vi "Operator Loop OLD.vi"() -> ()   [LabVIEW 2011]
uses:
  <vilib>/Platform/TimedLoop/XDataNode/timing_clust.ctl
  <vilib>/Platform/TimedLoop/XDataNode/nitl_modes.ctl
  <vilib>/Platform/TimedLoop/XDataNode/wakeup.ctl
  <vilib>/Platform/TimedLoop/XDataNode/XDataNode.xnode
  <vilib>/Platform/TimedLoop/XDataNode/XDNodeRunTimeDep.lvlib
panel:
  out "Heading_Cmd":dbl
  out "VTan_Cmd":dbl
  out "VAng_Cmd":dbl
  in  "End Loop":bool
  out "Error Out":errorcluster
  in  "Error In":errorcluster
  in  "SubGoal Threshold":dbl=1.1
  in  "GPS Data":T1
  in  "IMU Data":T2
  in  "A star":bool=TRUE
  in  "outer threshold":dbl=1.1
  in  "inner threshold":dbl=0.6
  in  "max speed":dbl=0.4
  in  "stop?":bool
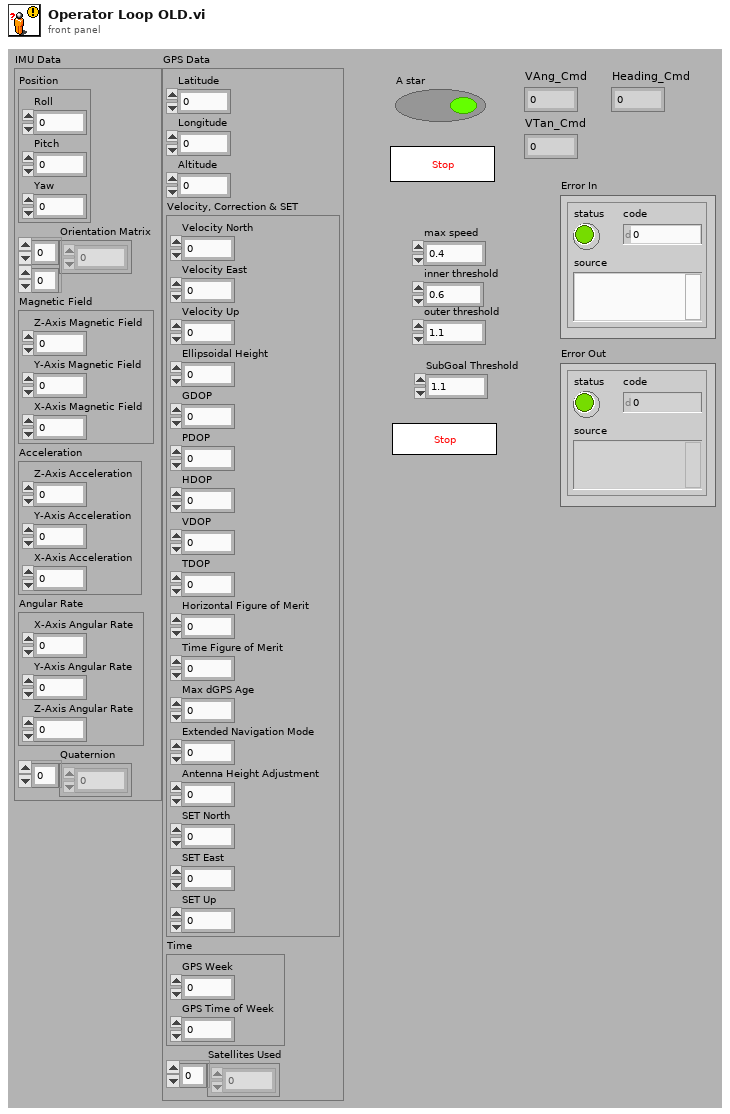
[diagram p1: front panel]
types:
  T1 = cluster{"Latitude":dbl, "Longitude":dbl, "Altitude":dbl, "Velocity, Correction & SET":cluster{"Velocity North":dbl, "Velocity East":dbl, "Velocity Up":dbl, "Ellipsoidal Height":dbl, "GDOP":sgl, "PDOP":sgl, "HDOP":sgl, "VDOP":sgl, "TDOP":sgl, "Horizontal Figure of Merit":u8, "Time Figure of Merit":u8, "Max dGPS Age":sgl, "Extended Navigation Mode":u8, "Antenna Height Adjustment ":dbl, "SET North":i32, "SET East":i32, "SET Up":i32}, "Time":cluster{"GPS Week":u16, "GPS Time of Week":sgl}, "Satellites Used":i32[]}
  T2 = cluster{"Position":cluster{"Roll":dbl, "Pitch":dbl, "Yaw":dbl}, "Orientation Matrix":dbl[][], "Magnetic Field":cluster{"Z-Axis Magnetic Field":dbl, "Y-Axis Magnetic Field":dbl, "X-Axis Magnetic Field":dbl}, "Acceleration":cluster{"Z-Axis Acceleration":dbl, "Y-Axis Acceleration":dbl, "X-Axis Acceleration":dbl}, "Angular Rate":cluster{"X-Axis Angular Rate":dbl, "Y-Axis Angular Rate":dbl, "Z-Axis Angular Rate":dbl}, "Quaternion":dbl[]}
  T3 = enum16{"Idle", "Wiimote", "Joypad", "IGVC", "Avoide Objects", "Avoide Lines", "Path Planning", "Heading", "Waypoint"}
  T4 = typedef "XDNodeRunTimeDep.lvlib/timing_clust.ctl" = cluster{"Expected End [f-1]":u64, "Actual End [f-1]":u64, "Finished Late? [f-1]":bool, "Expected End [i-1]":u64, "Actual End [i-1]":u64, "Finished Late? [i-1]":bool, "Expected Start [i]":u64, "Actual Start [i]":u64, "Expected Start [f]":u64, "Actual Start [f]":u64, "Source Name":string, "Structure Name":string, "Period":i64, "Deadline":i64, "Offset":i64, "Start":i64, "Priority":i32, "Timeout":i32, "Mode":T5, "Wakeup Reason":T6, "Error":errorcluster, "Source Type":string, "Secondary Source Type":string, "Global End Time":u64, "Global Start Time":u64, "Frame Duration":u64, "Iteration Duration":u64, "Assigned CPU":i32, "I/O Scan Engine Mode":u32}
  T5 = typedef "XDNodeRunTimeDep.lvlib/nitl_modes.ctl" = enum32{"No Change", "Process missed periods, maintain original phase", "Discard missed periods, maintain original phase", "Process missed periods, ignore original phase", "Discard missed periods, ignore original phase"}
  T6 = typedef "XDNodeRunTimeDep.lvlib/wakeup.ctl" = enum32{"Normal", "Aborted", "Asynchronous wakeup", "Timing source error", "Timed loop error", "Timeout"}
  T7 = cluster{"SubGoal":cluster{"Latitude":dbl, "Longitude":dbl, "Altitude":dbl, "Velocity, Correction & SET":cluster{"Velocity North":dbl, "Velocity East":dbl, "Velocity Up":dbl, "Ellipsoidal Height":dbl, "GDOP":sgl, "PDOP":sgl, "HDOP":sgl, "VDOP":sgl, "TDOP":sgl, "Horizontal Figure of Merit":u8, "Time Figure of Merit":u8, "Max dGPS Age":sgl, "Extended Navigation Mode":u8, "Antenna Height Adjustment ":dbl, "SET North":i32, "SET East":i32, "SET Up":i32}, "Time":cluster{"GPS Week":u16, "GPS Time of Week":sgl}, "Satellites Used":i32[]}, "Sub Goal Name":string}[]
  T8 = cluster{"SubGoal":cluster{"Latitude":dbl, "Longitude":dbl, "Altitude":dbl, "Velocity, Correction & SET":cluster{"Velocity North":dbl, "Velocity East":dbl, "Velocity Up":dbl, "Ellipsoidal Height":dbl, "GDOP":sgl, "PDOP":sgl, "HDOP":sgl, "VDOP":sgl, "TDOP":sgl, "Horizontal Figure of Merit":u8, "Time Figure of Merit":u8, "Max dGPS Age":sgl, "Extended Navigation Mode":u8, "Antenna Height Adjustment ":dbl, "SET North":i32, "SET East":i32, "SET Up":i32}, "Time":cluster{"GPS Week":u16, "GPS Time of Week":sgl}, "Satellites Used":i32[]}, "Sub Goal Name":string}
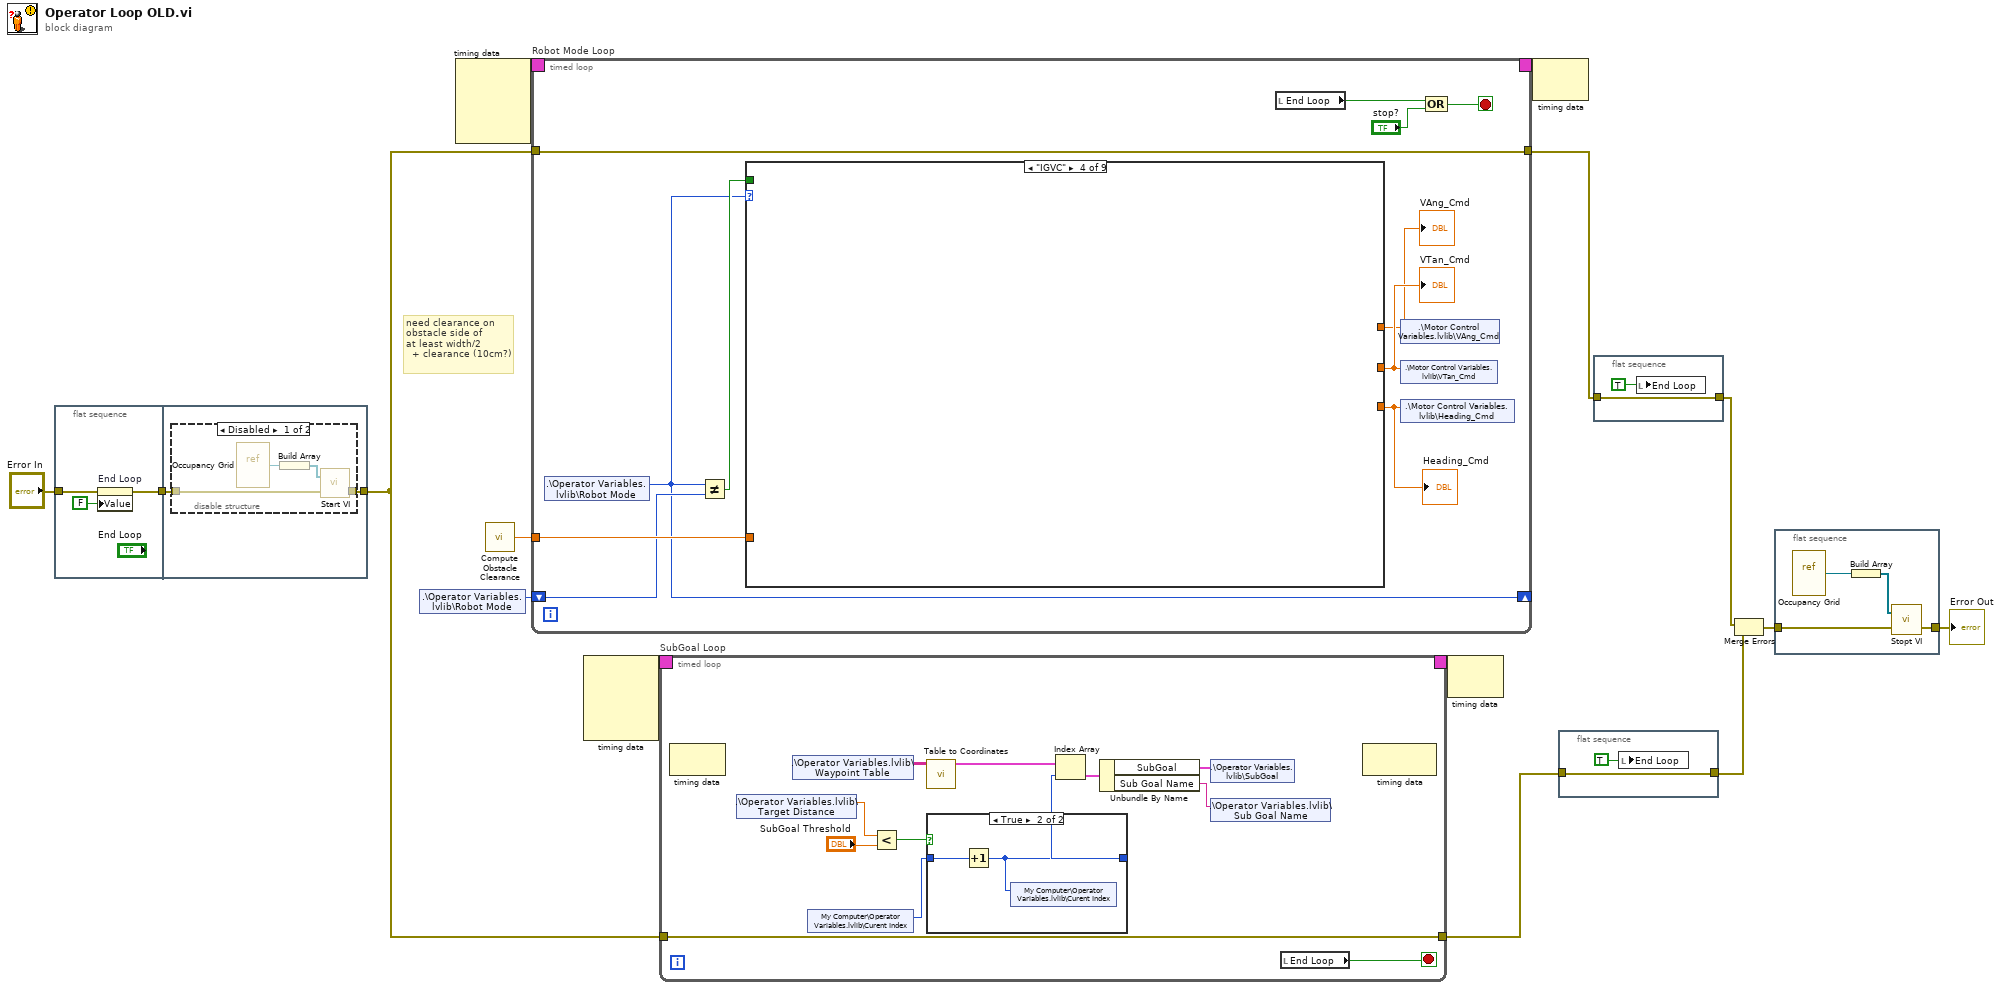
[diagram p0: block diagram]
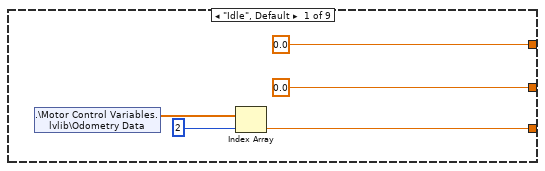
[diagram p4: hidden frame]
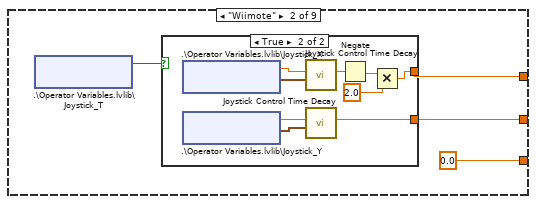
[diagram p5: hidden frame]
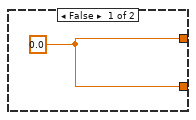
[diagram p6: hidden frame]
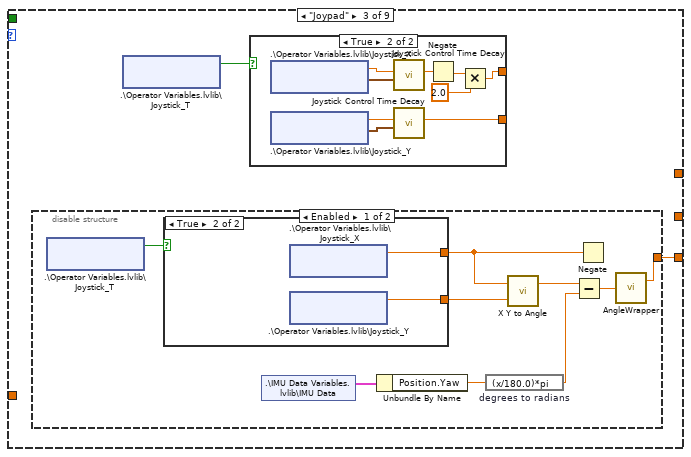
[diagram p7: hidden frame]
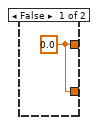
[diagram p8: hidden frame]
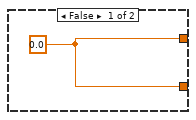
[diagram p10: hidden frame]
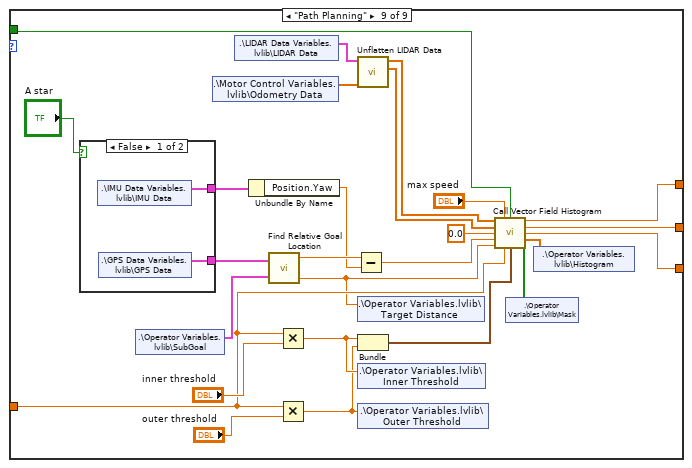
[diagram p15: hidden frame]
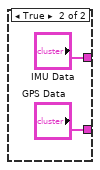
[diagram p16: hidden frame]
diagram:
  # "need clearance on \nobstacle side of \nat least width/2 \n  + clearance (10cm?)"
  n1 = flat-sequence {
    tunnel: "Error In" -> [w16]
    tunnel: [w17] -> w4
    tunnel: [w19] -> w5
    tunnel: w4 -> [w20]
    frame #0 {
      n2 = property on="End Loop" class="Bool (strict)"(error in=w16, "Value"=FALSE ("End Loop")) -> (error out=w17:errorcluster)  [unwired: 1 in, 1 out]
    }
    frame #1 {
      n3 = disable-structure shown="Disabled" {
        disable-tunnel: w20 -> [w22 w25]
        disable-tunnel: [w21 w25] -> w19
        frame Disabled {
          n4 = vi-ref "Occupancy Grid.vi"() -> (w24:refnum<vi>)
          n5 = Build Array(w24) -> (w23:refnum<vi>[])
          n6 = call "Start VI.vi"("error in"=w22, "VI refnum"=w23) -> ("error out"=w21:errorcluster)  [unwired: 1 in]
        }
        frame Enabled {
        }
      }
    }
  }
  n7 = shared-variable ".\\Operator Variables.lvlib\\Robot Mode"() -> (w12:T3)  [unwired: 1 in, 1 out]
  n8 = node-c288() -> (w15:T4)  [unwired: 4 in]
  n9 = call "Compute Obstacle Clearance.vi"() -> ("obstacle clearance (m)"=w13:dbl)  [unwired: 1 in]
  n10 = timed-loop "Robot Mode Loop" {
    timing: w15 -> [_]
    timing-out: [_] -> w14
    tunnel: w13 -> [w36]
    shift-right: [w33] -> _
    shift-left: w12 -> [w34]
    tunnel: w5 -> [w32]
    tunnel: [w32] -> w1
    stop <- w29 stop-if-true
    n11 = shared-variable ".\\Operator Variables.lvlib\\Robot Mode"() -> (w33:T3)  [unwired: 1 in, 1 out]
    n12 = Not Equal?(x=w33, y=w34) -> (x != y?=w35:bool)
    n13 = case shown="\"IGVC\"" w33 {
      tunnel: w36 -> [_ _ _ _ _ _ _ _ w98]
      tunnel: [w37 0.0 ("command vy") w56 _ _ _ _ _ w97] -> w28
      tunnel: [0.0 ("Double") w43 _ _ _ _ _ _ w91] -> w27
      tunnel: [0.0 w42 _ _ _ _ _ _ w92] -> w26
      tunnel: w35 -> [_ _ _ _ _ _ _ _ w103]
      frame "Idle", Default {
        n14 = shared-variable ".\\Motor Control Variables.lvlib\\Odometry Data"() -> (w39:dbl[])  [unwired: 1 in, 1 out]
        n15 = Index Array(array=w39, index=2) -> (element=w37:dbl)
      }
      frame "Wiimote" {
        n16 = shared-variable ".\\Operator Variables.lvlib\\Joystick_T"() -> (w45:bool)  [unwired: 1 in, 2 out]
        n17 = case shown="True" w45 {
          tunnel: [w46 w51] -> w43
          tunnel: [w46 w48] -> w42
          frame False {
            w46 = 0.0
          }
          frame True {
            n18 = shared-variable ".\\Operator Variables.lvlib\\Joystick_X"() -> (w55:dbl, w54:timestamp)  [unwired: 1 in, 1 out]
            n19 = shared-variable ".\\Operator Variables.lvlib\\Joystick_Y"() -> (w52:dbl, w53:timestamp)  [unwired: 1 in, 1 out]
            n20 = call "Joystick Control Time Decay.vi"("Value"=w55, "Time Stamp"=w54) -> ("Decayed Value"=w50:dbl)  [unwired: 8 in]
            n21 = call "Joystick Control Time Decay.vi"("Value"=w52, "Time Stamp"=w53) -> ("Decayed Value"=w51:dbl)  [unwired: 8 in]
            n22 = Negate(x=w50) -> (-x=w49:dbl)
            n23 = Multiply(x=w49, y=2.0) -> (x*y=w48:dbl)
          }
        }
      }
      frame "Joypad" {
        n24 = disable-structure shown="Enabled" {
          disable-tunnel: [w58 _] -> w56
          frame Enabled {
            n25 = shared-variable ".\\Operator Variables.lvlib\\Joystick_T"() -> (w66:bool)  [unwired: 1 in, 2 out]
            n26 = case shown="True" w66 {
              tunnel: [w67 w68] -> w63
              tunnel: [w67 w69] -> w64
              frame False {
                w67 = 0.0
              }
              frame True {
                n27 = shared-variable ".\\Operator Variables.lvlib\\Joystick_X"() -> (w69:dbl)  [unwired: 1 in, 2 out]
                n28 = shared-variable ".\\Operator Variables.lvlib\\Joystick_Y"() -> (w68:dbl)  [unwired: 1 in, 2 out]
              }
            }
            n29 = shared-variable ".\\IMU Data Variables.lvlib\\IMU Data"() -> (w65:T2)  [unwired: 1 in, 1 out]
            n30 = Unbundle By Name(w65) -> ("Position.Yaw"=w62:dbl)
            n31 = expression code="(x/180.0)*pi" "degrees to radians"(w62) -> (w61:dbl)
            n32 = call "X Y to Angle.vi"("y"=w63, "x"=w64) -> ("Heading Out (rad)"=w60:dbl)  [unwired: 1 out]
            n33 = Subtract(x=w60, y=w61) -> (x-y=w59:dbl)
            n34 = Negate(x=w64) -> ()  [unwired: 1 out]
            n35 = call "AngleWrapper.vi"("Heading In (rad)"=w59) -> ("Heading Out (rad)"=w58:dbl)  [unwired: 1 out]
          }
          frame Disabled {
          }
        }
        n36 = shared-variable ".\\Operator Variables.lvlib\\Joystick_T"() -> (w57:bool)  [unwired: 1 in, 2 out]
        n37 = case shown="True" w57 {
          tunnel: [w70 w75] -> _
          tunnel: [w70 w72] -> _
          frame False {
            w70 = 0.0
          }
          frame True {
            n38 = shared-variable ".\\Operator Variables.lvlib\\Joystick_X"() -> (w79:dbl, w78:timestamp)  [unwired: 1 in, 1 out]
            n39 = shared-variable ".\\Operator Variables.lvlib\\Joystick_Y"() -> (w76:dbl, w77:timestamp)  [unwired: 1 in, 1 out]
            n40 = call "Joystick Control Time Decay.vi"("Value"=w79, "Time Stamp"=w78) -> ("Decayed Value"=w74:dbl)  [unwired: 8 in]
            n41 = call "Joystick Control Time Decay.vi"("Value"=w76, "Time Stamp"=w77) -> ("Decayed Value"=w75:dbl)  [unwired: 8 in]
            n42 = Negate(x=w74) -> (-x=w73:dbl)
            n43 = Multiply(x=w73, y=2.0) -> (x*y=w72:dbl)
          }
        }
      }
      frame "IGVC" {
      }
      frame "Avoide Objects" {
      }
      frame "Avoide Lines" {
      }
      frame "Heading" {
      }
      frame "Waypoint" {
      }
      frame "Path Planning" {
        n44 = case shown="False" "A star" {
          tunnel: [w107 "GPS Data"] -> w89
          tunnel: [w106 "IMU Data"] -> w86
          frame False {
            n45 = shared-variable ".\\IMU Data Variables.lvlib\\IMU Data"() -> (w106:T2)  [unwired: 1 in, 1 out]
            n46 = shared-variable ".\\GPS Data Variables.lvlib\\GPS Data"() -> (w107:T1)  [unwired: 1 in, 1 out]
          }
          frame True {
          }
        }
        n47 = shared-variable ".\\Operator Variables.lvlib\\SubGoal"() -> (w88:T1)  [unwired: 1 in, 1 out]
        n48 = shared-variable ".\\Motor Control Variables.lvlib\\Odometry Data"() -> (w87:dbl[])  [unwired: 1 in, 1 out]
        n49 = shared-variable ".\\LIDAR Data Variables.lvlib\\LIDAR Data"() -> (w90:cluster{"Magnitude":dbl[], "Direction":dbl[]})  [unwired: 1 in, 1 out]
        n50 = Unbundle By Name(w86) -> ("Position.Yaw"=w83:dbl)
        n51 = call "Find Relative Goal Location.vi"("Current Position"=w89, "Goal Position"=w88) -> ("Target Heading (deg)"=w84:dbl, "Target Distance"=w96:dbl)  [unwired: 1 out]
        n52 = Multiply(x=w98, y="inner threshold") -> (x*y=w95:dbl)
        n53 = Multiply(x=w98, y="outer threshold") -> (x*y=w94:dbl)
        n54 = Subtract(x=w84, y=w83) -> (x-y=w82:dbl)
        n55 = call "Unflatten LIDAR Data.vi"("Odometry Data"=w87, "LIDAR Data"=w90) -> ("Bearing (rad)"=w104:dbl[], "Range (m)"=w105:dbl[])  [unwired: 8 in]
        n56 = shared-variable ".\\Operator Variables.lvlib\\Target Distance"(w96) -> ()  [unwired: 1 in, 1 out]
        n57 = Bundle(w95, w94) -> (w93:cluster{dbl, dbl})  [unwired: 1 in]
        n58 = shared-variable ".\\Operator Variables.lvlib\\Inner Threshold"(w95) -> ()  [unwired: 1 in, 1 out]
        n59 = shared-variable ".\\Operator Variables.lvlib\\Outer Threshold"(w94) -> ()  [unwired: 1 in, 1 out]
        n60 = call "Call Vector Field Histogram.vi"("LIDAR magn. (m)"=w105, "max speed"="max speed", "Initialize?"=w103, "LIDAR angle (rad)"=w104, "current heading (rad)"=0.0, "target heading (rad)"=w82, "target distance"=w96, "obstacle clearance (m)"=w98, "thresholds"=w93) -> ("command vx"=w92:dbl, "command vy"=w91:dbl, "command heading (rad)"=w97:dbl, "histogram out"=w99:dbl[], "mask out"=w81:bool[])  [unwired: 2 in]
        n61 = shared-variable ".\\Operator Variables.lvlib\\Mask"(w81) -> ()  [unwired: 1 in, 1 out]
        n62 = shared-variable ".\\Operator Variables.lvlib\\Histogram"(w99) -> ()  [unwired: 1 in, 1 out]
      }
    }
    "VAng_Cmd" <- w26
    "VTan_Cmd" <- w27
    "Heading_Cmd" <- w28
    n63 = local read "End Loop"() -> (w30:bool)
    n64 = shared-variable ".\\Motor Control Variables.lvlib\\VAng_Cmd"(w26) -> ()  [unwired: 1 in, 1 out]
    n65 = shared-variable ".\\Motor Control Variables.lvlib\\VTan_Cmd"(w27) -> ()  [unwired: 1 in, 1 out]
    n66 = shared-variable ".\\Motor Control Variables.lvlib\\Heading_Cmd"(w28) -> ()  [unwired: 1 in, 1 out]
    n67 = Compound Arithmetic op=OR(w30, "stop?") -> (w29:bool)
  }
  n68 = node-c288() -> (w11:T4)  [unwired: 4 in]
  n69 = timed-loop "SubGoal Loop" {
    timing: w11 -> [_]
    timing-out: [_] -> w10
    tunnel: w5 -> [w116]
    tunnel: [w116] -> w7
    stop <- w115 stop-if-true
    n70 = node-c288() -> ()  [unwired: 1 in, 1 out]
    n71 = shared-variable ".\\Operator Variables.lvlib\\Target Distance"() -> (w123:dbl)  [unwired: 1 in, 1 out]
    n72 = shared-variable ".\\Operator Variables.lvlib\\Waypoint Table"() -> (w117:string[][])  [unwired: 1 in, 1 out]
    n73 = shared-variable "My Computer\\Operator Variables.lvlib\\Curent Index"() -> (w113:i32)  [unwired: 1 in, 1 out]
    n74 = Less?(x=w123, y="SubGoal Threshold") -> (x < y?=w114:bool)
    n75 = call "Table to Coordinates.vi"("Waypoint Table"=w117) -> ("Coordinates"=w118:T7)  [unwired: 10 in]
    n76 = case shown="True" w114 {
      tunnel: w113 -> [w124 w126]
      tunnel: [w124 w125] -> w112
      frame False {
      }
      frame True {
        n77 = Increment(x=w126) -> (x+1=w125:i32)
        n78 = shared-variable "My Computer\\Operator Variables.lvlib\\Curent Index"(w125) -> ()  [unwired: 1 in, 1 out]
      }
    }
    n79 = Index Array(array=w118, index=w112) -> (element=w119:T8)
    n80 = Unbundle By Name(w119) -> ("SubGoal"=w120:T1, "Sub Goal Name"=w121:string)
    n81 = shared-variable ".\\Operator Variables.lvlib\\SubGoal"(w120) -> ()  [unwired: 1 in, 1 out]
    n82 = shared-variable ".\\Operator Variables.lvlib\\Sub Goal Name"(w121) -> ()  [unwired: 1 in, 1 out]
    n83 = local read "End Loop"() -> (w115:bool)
    n84 = node-c288() -> ()  [unwired: 1 in, 1 out]
  }
  n85 = node-c288(w10) -> ()  [unwired: 1 out]
  n86 = node-c288(w14) -> ()  [unwired: 1 out]
  n87 = flat-sequence {
    tunnel: w7 -> [w129]
    tunnel: [w129] -> w9
    frame #0 {
      n88 = local write "End Loop"(TRUE ("End Loop")) -> ()
    }
  }
  n89 = flat-sequence {
    tunnel: [w131] -> w8
    tunnel: w1 -> [w131]
    frame #0 {
      n90 = local write "End Loop"(TRUE ("End Loop")) -> ()
    }
  }
  n91 = Merge Errors(w8, w9) -> (w2:errorcluster)
  n92 = flat-sequence {
    tunnel: [w133] -> w3
    tunnel: w2 -> [w134]
    frame #0 {
      n93 = vi-ref "Occupancy Grid.vi"() -> (w135:refnum<vi>)
      n94 = Build Array(w135) -> (w136:refnum<vi>[])
      n95 = call "Stopt VI.vi"("error in"=w134, "VI refnum"=w136) -> ("error out"=w133:errorcluster)  [unwired: 1 in]
    }
  }
  "Error Out" <- w3
